vi "MovePosition_Primitive.vi"(0 "Side":T2, 1 "node":string, 2 "Arm Angles (degrees)":T1, 3 "error in":errorcluster) -> (6 "error out":errorcluster)   [LabVIEW 2013]
uses:
  ROS/Code/SubVIs/BaxterSide.ctl
  ROS/Code/SubVIs/BaxterArmsSmall.ctl
  Command_Joint_Angles_cluster.vi
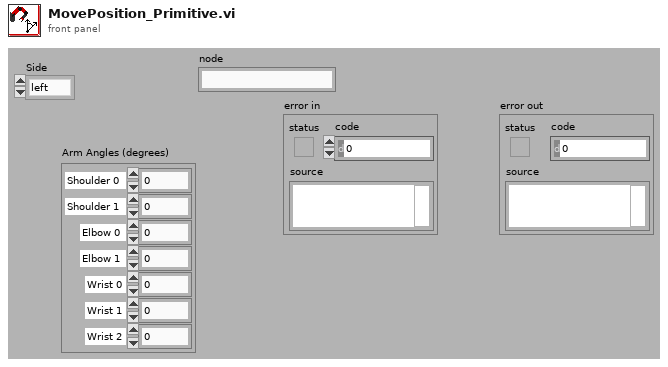
[diagram p1: front panel]
types:
  T1 = typedef "BaxterArmsSmall.ctl" = cluster{"Elbow 0":dbl, "Elbow 1":dbl, "Shoulder 0":dbl, "Shoulder 1":dbl, "Wrist 0":dbl, "Wrist 1":dbl, "Wrist 2":dbl}
  T2 = typedef "BaxterSide.ctl" = enum16{"left", "right"}
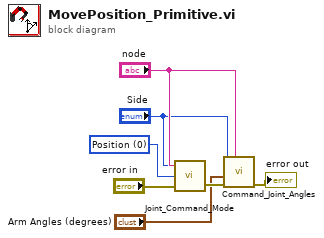
[diagram p0: block diagram]
diagram:
  w6 = u8 0 items=["Position", "Velocity", "Effort"] ("Mode")
  n1 = call "Joint_Command_Mode.vi"("Side"="Side", "node"="node", "Mode"=w6, "error in"="error in") -> ("error out"=w7:errorcluster)  [unwired: 2 in]
  n2 = call-poly "Command_Joint_Angles.vi"("node"="node", "error in"=w7, "Arm Angles (degrees)"="Arm Angles (degrees)", "Side"="Side") -> ("error out"=→"error out":errorcluster)  [unwired: 5 in]
